vi "PeltierPID_FinalDesign_AR_edits.vi"() -> ()   [LabVIEW 2019]
uses:
  <vilib>/Utility/error.llb/DialogType.ctl
  <vilib>/DAQmx/write.llb/DAQmx Write (Digital Bool 1Line 1Point).vi
  <vilib>/DAQmx/read.llb/DAQmx Read (Analog DBL 1Chan 1Samp).vi
  <vilib>/Analysis/baseanly.llb/Mean (DBL).vi
  <vilib>/DAQmx/create/channels.llb/DAQmx Create Channel (DO-Digital Output).vi
  <vilib>/DAQmx/miscellaneous.llb/DAQmx Fill In Error Info.vi
  PeltierPID_FinalDesignFeb2022/Global 5.vi
  <instrlib>/BK Precision 178XB Series/BK Precision 178XB Series.lvlib
  <vilib>/Analysis/NI_AALBase.lvlib
panel:
  out "Integrated error":dbl
  out "Line(s)":tag="Dev3/port0/line1"
  out "Rude Temp":dbl format="%0.2f"
  out "averageTemperature":dbl[](array[numeric])
  out "overshoot_threshold":dbl
  out "Output Voltage":dbl
  in  "dt ( -1 is default)":dbl=-1.0 format="%.3f"
  in  "setpoint":dbl format="%.2f"
  out "temp. Graph":dbl(graph)
  out "Output voltage Graph":dbl(graph)
  in  "?":bool
  out "Reak-time voltage":dbl format="%.2f"
  out "Thermocouple":dbl
  in  "Current Limit (3 A)":dbl min=0.0 max=6.0 format="%#.2g"
  in  "Maximum Output Voltage (18)":dbl=18.0 min=0.0 max=72.0 format="%#.2f"
  in  "VISA resource name":refnum<visa-resource-name>
  out "Polarity Boolean":bool
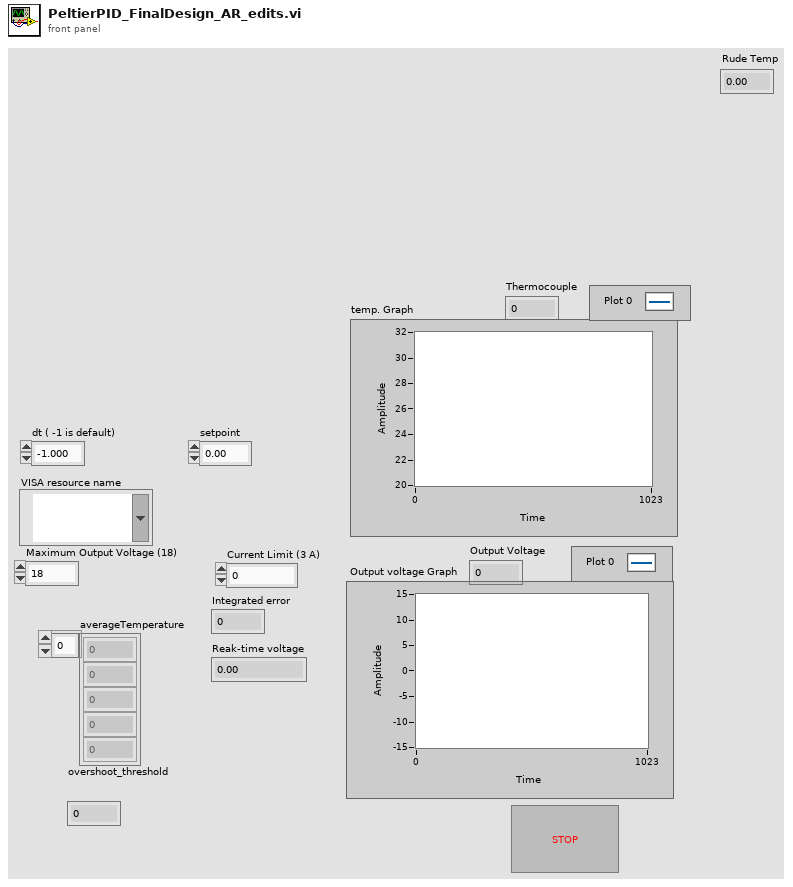
[diagram p1: front panel]
types:
  T1 = cluster{"proportional gain (Kc)":dbl, "integral time (Ti, min)":dbl, "derivative time (Td, min)":dbl}
  T2 = typedef "DialogType.ctl" = u16
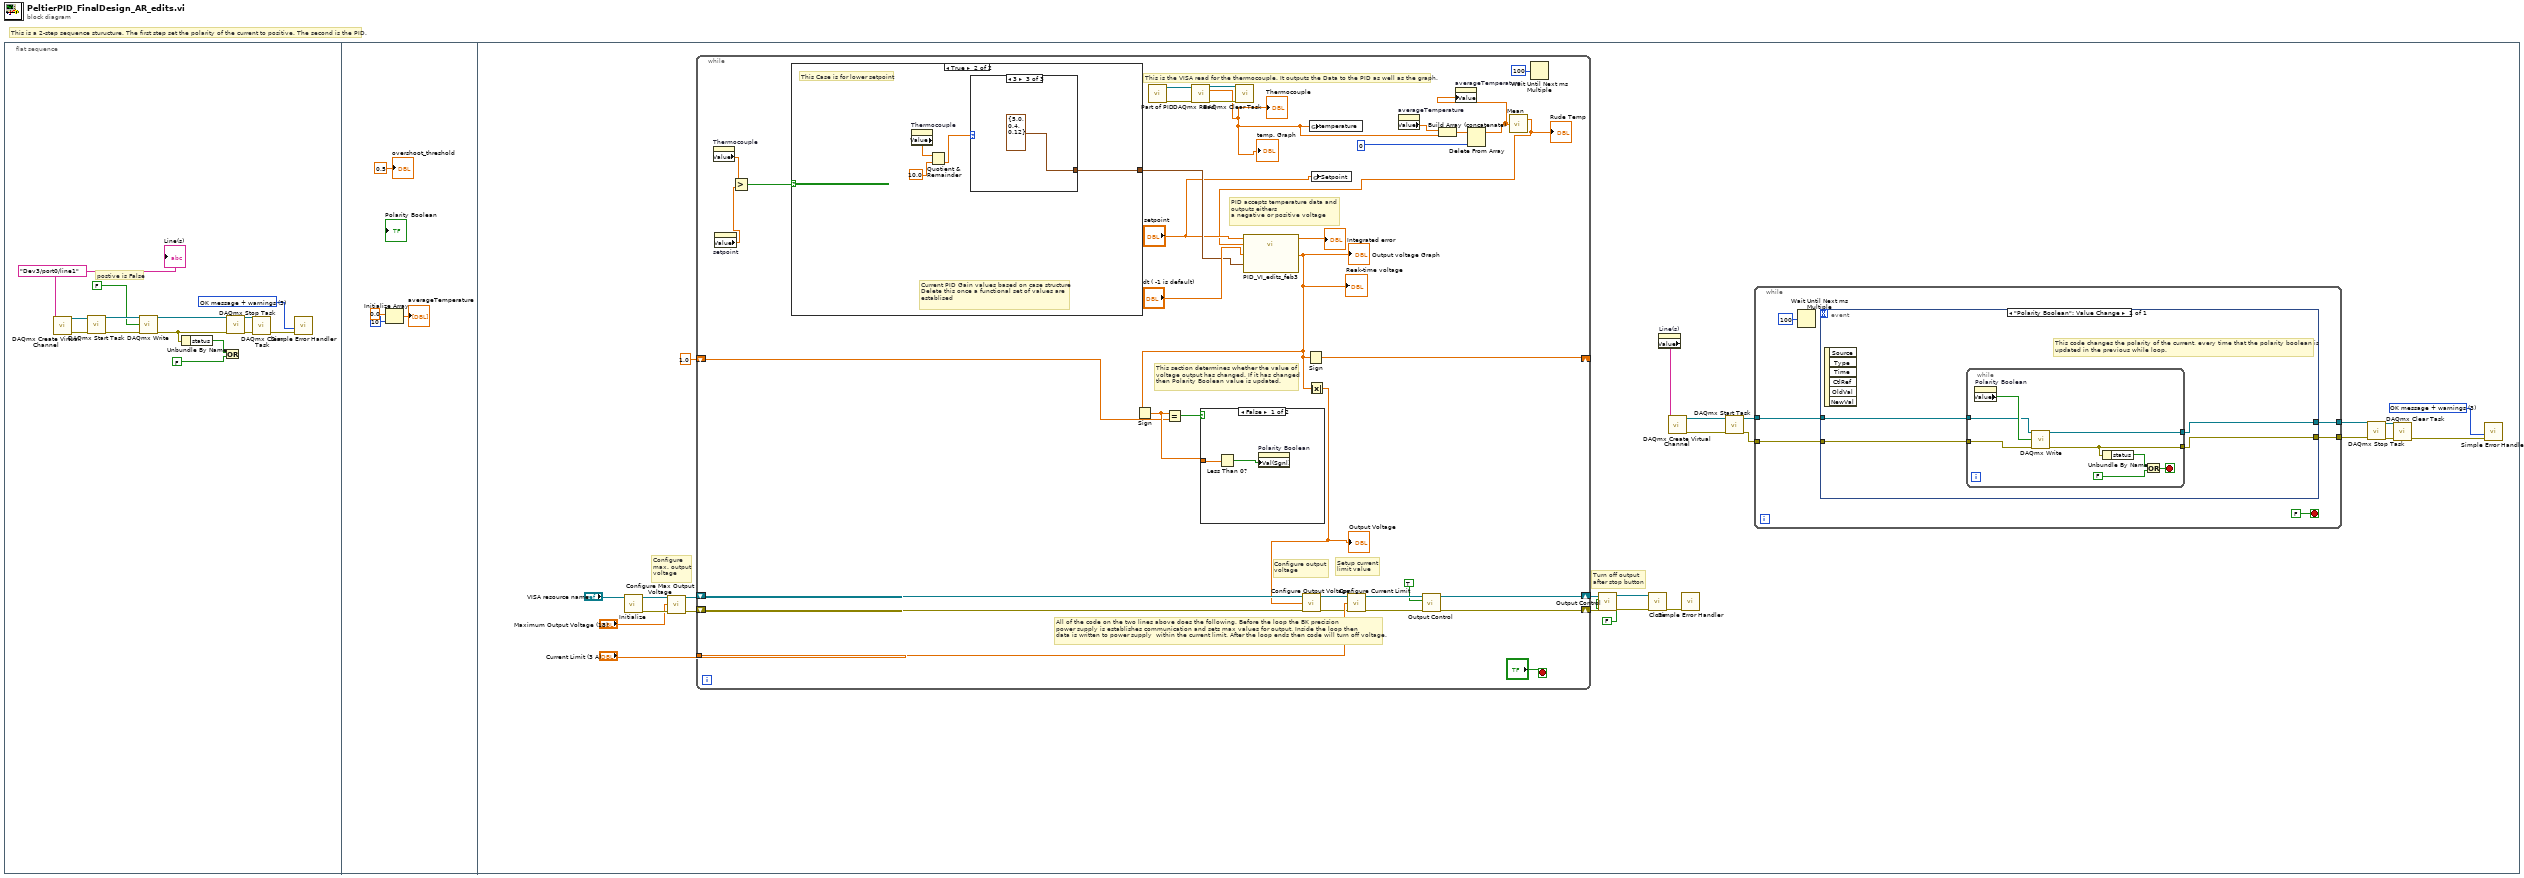
[diagram p0: block diagram]
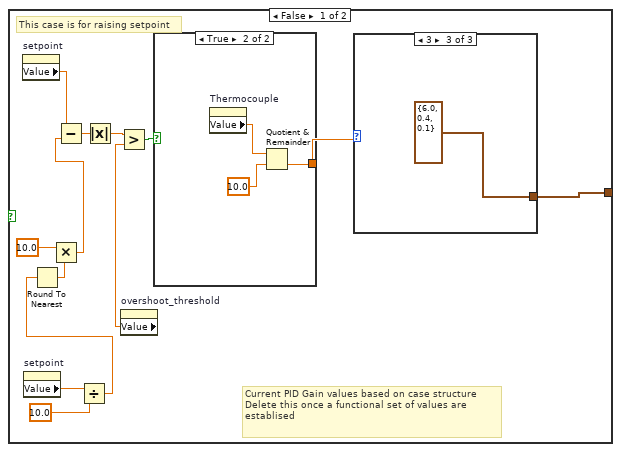
[diagram p2: hidden frame]
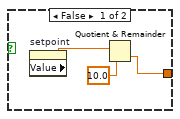
[diagram p3: hidden frame]
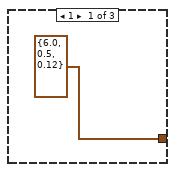
[diagram p4: hidden frame]
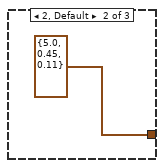
[diagram p5: hidden frame]
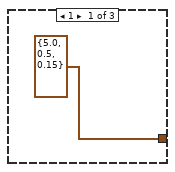
[diagram p6: hidden frame]
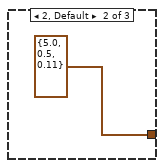
[diagram p7: hidden frame]
diagram:
  # "This is a 2-step sequence sturucture. The first step set the polarity of the current to positive. The second is the PID."
  n1 = flat-sequence {
    frame #0 {
      w7 = tag "Dev3/port0/line1" ("Line(s)")
      w14 = T2 3 items=["no dialog", "OK message", "continue or stop message", "OK message + warnings", "continue/stop + warnings"] ("type of dialog (OK msg:1)")
      # "postive is False"
      n2 = call-poly <vilib>:"DAQmx Create Virtual Channel.vi"("lines"=w7) -> ("task out"=w9:refnum<k21>, "error out"=w8:errorcluster)  [unwired: 13 in]
      n3 = call <vilib>:"DAQmx Start Task.vi"("task/channels in"=w9, "error in"=w8) -> ("task out"=w4:refnum<k21>, "error out"=w5:errorcluster)  [unwired: 12 in]
      n4 = call-poly <vilib>:"DAQmx Write.vi"("task/channels in"=w4, "data"=FALSE ("Reverse Polarity"), "error in"=w5) -> ("task out"=w12:refnum<k21>, "error out"=w13:errorcluster)  [unwired: 10 in, 1 out]
      n5 = Unbundle By Name(w13) -> ("status"=w3:bool)
      n6 = Or(x=w3, y=FALSE ("Stop")) -> ()  [unwired: 1 out]
      n7 = call <vilib>:"DAQmx Stop Task.vi"("task/channels in"=w12, "error in"=w13) -> ("task out"=w10:refnum<k21>, "error out"=w11:errorcluster)  [unwired: 12 in]
      n8 = call <vilib>:"DAQmx Clear Task.vi"("task in"=w10, "error in"=w11) -> ("error out"=w6:errorcluster)  [unwired: 13 in]
      n9 = call <vilib>:"Simple Error Handler.vi"("type of dialog (OK msg:1)"=w14, "error in (no error)"=w6) -> ()  [unwired: 3 in, 5 out]
      "Line(s)" <- w7
    }
    frame #1 {
      n10 = Initialize Array(0.0 ("element"), 10 ("dimension size")) -> (→"averageTemperature":dbl[])
      "overshoot_threshold" <- 0.5 ("Numeric")
    }
    frame #2 {
      w19 = T2 3 items=["no dialog", "OK message", "continue or stop message", "OK message + warnings", "continue/stop + warnings"] ("type of dialog (OK msg:1)")
      # "Turn off output\nafter stop button"
      # "Configure\nmax. output\nvoltage"
      n11 = call "Initialize.vi"("VISA resource name"="VISA resource name") -> ("error out"=w36:errorcluster, "VISA resource name out"=w35:refnum<visa-resource-name>)  [unwired: 9 in]
      n12 = call "Configure Max Output Voltage.vi"("VISA resource name"=w35, "Maximum Output Voltage (18)"="Maximum Output Voltage (18)", "error in (no error)"=w36) -> ("VISA resource name out"=w37:refnum<visa-resource-name>, "error out"=w38:errorcluster)  [unwired: 11 in]
      n13 = while {
        tunnel: "Current Limit (3 A)" -> [w96]
        shift-right: [w93] -> w40
        shift-left: w37 -> [w95]
        shift-right: [w92] -> w41
        shift-left: w38 -> [w94]
        shift-right: [w80] -> _
        shift-left: 1.0 -> [w79]
        stop <- "?" stop-if-true
        # "All of the code on the two lines above does the following. Before the loop the BK precision \npower supply is establishes communication and sets max values for output. Inside the loop then \ndata is written to power supply  within the current limit. After the loop ends then code will turn off voltage."
        # "This section determines whether the value of \nvoltage output has changed. If it has changed \nthen Polarity Boolean value is updated."
        # "PID accepts temperature data and outputs eithers \na negative or positive voltage"
        # "This is the VISA read for the thermocouple. It outputs the Data to the PID as well as the graph."
        # "Setup current\nlimit value"
        # "Configure output\nvoltage"
        n14 = property on="Thermocouple" class="DigNum (strict)"() -> ("Value"=w74:dbl)  [unwired: 2 in, 2 out]
        n15 = property on="setpoint" class="DigNum (strict)"() -> ("Value"=w73:dbl)  [unwired: 2 in, 2 out]
        n16 = Greater?(x=w74, y=w73) -> (0:w75:bool)
        n17 = case shown="True" w75 {
          tunnel: [w109 w119] -> w71
          frame False {
            # "This case is for raising setpoint"
            # "Current PID Gain values based on case structure\nDelete this once a functional set of values are establised"
            n18 = property on="setpoint" class="DigNum (strict)"() -> ("Value"=w104:dbl)  [unwired: 2 in, 2 out]
            n19 = property on="setpoint" class="DigNum (strict)"() -> ("Value"=w103:dbl)  [unwired: 2 in, 2 out]
            n20 = Divide(x=w103, y=10.0) -> (x/y=w101:dbl)
            n21 = Round To Nearest(number=w101) -> (nearest integer value=w100:dbl)
            n22 = Multiply(x=10.0, y=w100) -> (x*y=w98:dbl)
            n23 = Subtract(x=w104, y=w98) -> (x-y=w106:dbl)
            n24 = Absolute Value(x=w106) -> (abs(x)=w107:dbl)
            n25 = property on="overshoot_threshold" class="DigNum (strict)"() -> ("Value"=w97:dbl)  [unwired: 2 in, 2 out]
            n26 = Greater?(x=w107, y=w97) -> (0:w108:bool)
            n27 = case shown="True" w108 {
              tunnel: [w110 w113] -> w105
              frame False {
                n28 = property on="setpoint" class="DigNum (strict)"() -> ("Value"=w112:dbl)  [unwired: 2 in, 2 out]
                n29 = Quotient & Remainder(x=w112, y=10.0) -> (floor(x/y)=w110:dbl)  [unwired: 1 out]
              }
              frame True {
                n30 = property on="Thermocouple" class="DigNum (strict)"() -> ("Value"=w115:dbl)  [unwired: 2 in, 2 out]
                n31 = Quotient & Remainder(x=w115, y=10.0) -> (floor(x/y)=w113:dbl)  [unwired: 1 out]
              }
            }
            n32 = case shown="3" w105 {
              tunnel: [T1 {"proportional gain (Kc)"=6.0, "integral time (Ti, min)"=0.5, "derivative time (Td, min)"=0.12} ("PID Gain Values") T1 {"proportional gain (Kc)"=5.0, "integral time (Ti, min)"=0.45, "derivative time (Td, min)"=0.11} ("PID Gain Values") T1 {"proportional gain (Kc)"=6.0, "integral time (Ti, min)"=0.4, "derivative time (Td, min)"=0.1} ("PID Gain Values")] -> w109
              frame 1 {
              }
              frame 2, Default {
              }
              frame 3 {
              }
            }
          }
          frame True {
            # "This Case is for lower setpoint"
            # "Current PID Gain values based on case structure\nDelete this once a functional set of values are establised"
            n33 = property on="Thermocouple" class="DigNum (strict)"() -> ("Value"=w122:dbl)  [unwired: 2 in, 2 out]
            n34 = Quotient & Remainder(x=w122, y=10.0) -> (floor(x/y)=w120:dbl)  [unwired: 1 out]
            n35 = case shown="3" w120 {
              tunnel: [T1 {"proportional gain (Kc)"=5.0, "integral time (Ti, min)"=0.5, "derivative time (Td, min)"=0.15} ("PID Gain Values") T1 {"proportional gain (Kc)"=5.0, "integral time (Ti, min)"=0.5, "derivative time (Td, min)"=0.11} ("PID Gain Values") T1 {"proportional gain (Kc)"=5.0, "integral time (Ti, min)"=0.4, "derivative time (Td, min)"=0.12} ("PID Gain Values")] -> w119
              frame 1 {
              }
              frame 2, Default {
              }
              frame 3 {
              }
            }
          }
        }
        n36 = call "Part of PID.vi"() -> ("error out"=w82:errorcluster, "task out"=w83:refnum<k21>)  [unwired: 10 in]
        n37 = call-poly <vilib>:"DAQmx Read.vi"("task/channels in"=w83, "error in"=w82) -> ("task out"=w84:refnum<k21>, "data"=w64:dbl, "error out"=w85:errorcluster)  [unwired: 11 in]
        "temp. Graph" <- w64
        "Thermocouple" <- w64
        n38 = call <vilib>:"DAQmx Clear Task.vi"("task in"=w84, "error in"=w85) -> ()  [unwired: 13 in, 1 out]
        n39 = global write "Global 5.vi" "temperature"(w64) -> ()
        n40 = global write "Global 5.vi" "Setpoint"("setpoint") -> ()
        n41 = property on="averageTemperature" class="Arr (strict)"() -> ("Value"=w67:dbl[])  [unwired: 2 in, 2 out]
        n42 = Build Array (concatenate)(w67, w64) -> (w69:dbl[])
        n43 = Delete From Array(array=w69, index=0) -> (array with subset deleted=w66:dbl[])  [unwired: 1 in, 1 out]
        n44 = property on="averageTemperature" class="Arr (strict)"("Value"=w66) -> ()  [unwired: 2 in, 2 out]
        n45 = call-poly <vilib>:"Mean.vi"("X"=w66) -> ("mean"=w65:dbl)  [unwired: 1 out]
        "Rude Temp" <- w65
        n46 = call "PID_VI_edits_feb3.vi"("PID gains"=w71, "dt (s)"="dt ( -1 is default)", "process variable"=w65, "setpoint"="setpoint") -> ("output"=w63:dbl, "Integrated error"=→"Integrated error":dbl)  [unwired: 5 in, 1 out]
        "Output voltage Graph" <- w63
        "Reak-time voltage" <- w63
        n47 = Sign(1:w63) -> (0:w81:dbl)
        n48 = Equal?(x=w81, y=w79) -> (x = y?=w76:bool)
        n49 = case shown="False" w76 {
          tunnel: w81 -> [w126 _]
          frame False {
            n50 = Less Than 0?(x=w126) -> (x < 0?=w127:bool)
            n51 = property on="Polarity Boolean" class="Bool (strict)"("Val(Sgnl)"=w127) -> ()  [unwired: 2 in, 2 out]
          }
          frame True {
          }
        }
        n52 = Sign(1:w63) -> (0:w80:dbl)
        n53 = Absolute Value(x=w63) -> (abs(x)=w77:dbl)
        "Output Voltage" <- w77
        n54 = call "Configure Output Voltage.vi"("VISA resource name"=w95, "Output Voltage (0)"=w77, "error in (no error)"=w94) -> ("VISA resource name out"=w91:refnum<visa-resource-name>, "error out"=w90:errorcluster)  [unwired: 11 in]
        n55 = call "Configure Current Limit.vi"("VISA resource name"=w91, "Current Limit (0)"=w96, "error in (no error)"=w90) -> ("VISA resource name out"=w89:refnum<visa-resource-name>, "error out"=w88:errorcluster)  [unwired: 11 in]
        n56 = call "Output Control.vi"("error in (no error)"=w88, "Enable Output Terminals (F: Off)"=TRUE, "VISA resource name"=w89) -> ("error out"=w92:errorcluster, "VISA resource name out"=w93:refnum<visa-resource-name>)  [unwired: 7 in]
        n57 = Wait Until Next ms Multiple(millisecond multiple=u32 100) -> ()  [unwired: 1 out]
      }
      n58 = call "Output Control.vi"("error in (no error)"=w41, "Enable Output Terminals (F: Off)"=FALSE, "VISA resource name"=w40) -> ("error out"=w43:errorcluster, "VISA resource name out"=w42:refnum<visa-resource-name>)  [unwired: 7 in]
      n59 = call "Close.vi"("error in (no error)"=w43, "VISA resource name"=w42) -> ("error out"=w39:errorcluster)  [unwired: 9 in]
      n60 = property on="Line(s)" class="DAQmxName"() -> ("Value"=w29:string)  [unwired: 2 in, 2 out]
      n61 = call-poly <vilib>:"DAQmx Create Virtual Channel.vi"("lines"=w29) -> ("task out"=w27:refnum<k21>, "error out"=w28:errorcluster)  [unwired: 13 in]
      n62 = call <vilib>:"Simple Error Handler.vi"("error in (no error)"=w39) -> ()  [unwired: 4 in, 5 out]
      n63 = call <vilib>:"DAQmx Start Task.vi"("task/channels in"=w27, "error in"=w28) -> ("task out"=w26:refnum<k21>, "error out"=w25:errorcluster)  [unwired: 12 in]
      n64 = while {
        tunnel: w26 -> [w47]
        tunnel: w25 -> [w46]
        tunnel: [w45] -> w21
        tunnel: [w44] -> w20
        stop <- FALSE stop-if-true
        n65 = Wait Until Next ms Multiple(millisecond multiple=u32 100) -> ()  [unwired: 1 out]
        n66 = event shown="[0] \"Polarity Boolean\": Value Change" {
          selector: _ -> [_]
          dyn-events: _ -> [_]
          timeout: _ -> [_]
          tunnel: w47 -> [w53]
          tunnel: w46 -> [w52]
          tunnel: [w51] -> w45
          tunnel: [w50] -> w44
          event "Polarity Boolean": Value Change {
            # "This code changes the polarity of the current, every time that the polarity boolean is \nupdated in the previous while loop."
            n67 = event-data() -> ()  [unwired: 1 in, 6 out]
            n68 = while {
              tunnel: [w59] -> w50
              tunnel: [w60] -> w51
              tunnel: w53 -> [w55]
              tunnel: w52 -> [w54]
              stop <- w61 stop-if-true
              n69 = property on="Polarity Boolean" class="Bool (strict)"() -> ("Value"=w56:bool)  [unwired: 2 in, 2 out]
              n70 = call-poly <vilib>:"DAQmx Write.vi"("task/channels in"=w55, "data"=w56, "error in"=w54) -> ("task out"=w60:refnum<k21>, "error out"=w59:errorcluster)  [unwired: 10 in, 1 out]
              n71 = Unbundle By Name(w59) -> ("status"=w58:bool)
              n72 = Or(x=w58, y=FALSE ("Stop")) -> (x .or. y?=w61:bool)
            }
          }
        }
      }
      n73 = call <vilib>:"DAQmx Stop Task.vi"("task/channels in"=w21, "error in"=w20) -> ("task out"=w23:refnum<k21>, "error out"=w24:errorcluster)  [unwired: 12 in]
      n74 = call <vilib>:"DAQmx Clear Task.vi"("task in"=w23, "error in"=w24) -> ("error out"=w22:errorcluster)  [unwired: 13 in]
      n75 = call <vilib>:"Simple Error Handler.vi"("type of dialog (OK msg:1)"=w19, "error in (no error)"=w22) -> ()  [unwired: 3 in, 5 out]
    }
  }
